vi "Keithley 27XX Finite Multi Read 1.vi"(0 "VISA resource name":refnum<visa-resource-name>, 5 "Channel List (101:110)":string="106,121", 7 "Sample Count (100)":i32=2, 11 "error in (no error)":errorcluster) -> (6 "Measurement Data":dbl[](array[numeric]), 15 "error out":errorcluster)   [LabVIEW 2015]
doc: "This example VI allows you to return an array of data from specifed channels.\n\nNote:\nFor front panel measurements, make sure the Input switch is in the out position(F)\nFor plug-in card measurements, make sure the Input switch is in the in poisition(R)"
uses:
  <instrlib>/Keithley 27XX/Public/Data/Read Multiple Direct.vi
  <instrlib>/Keithley 27XX/Keithley 27XX.lvlib
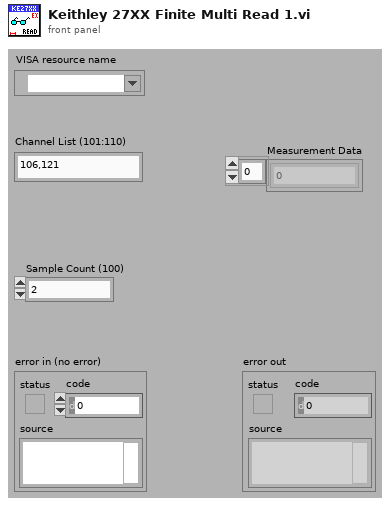
[diagram p1: front panel]
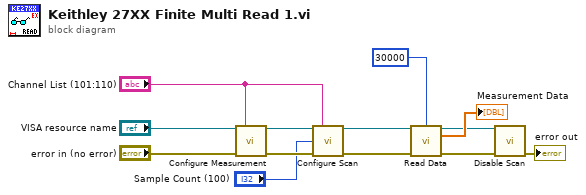
[diagram p0: block diagram]
diagram:
  n1 = call <instrlib>:"Configure Measurement.vi"("VISA resource name"="VISA resource name", "Scan List (Empty)"="Channel List (101:110)", "error in (no error)"="error in (no error)") -> ("VISA resource name out"=w13:refnum<visa-resource-name>, "error out"=w12:errorcluster)  [unwired: 11 in]
  n2 = call <instrlib>:"Configure Scan.vi"("VISA resource name"=w13, "Channel List (101:110)"="Channel List (101:110)", "Sample Count (100)"="Sample Count (100)", "error in (no error)"=w12) -> ("VISA resource name out"=w9:refnum<visa-resource-name>, "error out"=w10:errorcluster)  [unwired: 10 in]
  n3 = call-poly <instrlib>:"Read Data.vi"("VISA resource name"=w9, "Timeout (30000 milliseconds)"=u32 30000, "error in (no error)"=w10) -> ("VISA resource name out"=w4:refnum<visa-resource-name>, "Measurement Data"=→"Measurement Data":dbl[], "error out"=w5:errorcluster)  [unwired: 7 in, 3 out]
  n4 = call <instrlib>:"Disable Scan.vi"("VISA resource name"=w4, "error in (no error)"=w5) -> ("error out"=→"error out":errorcluster)  [unwired: 12 in, 1 out]
